vi "Simple Add.vi"(9 "Z":dbl, 10 "Y":dbl, 11 "X":dbl) -> (3 "Answer":dbl)   [LabVIEW 2016]
panel:
  # "Answer = 2x(X+Y+Z)"
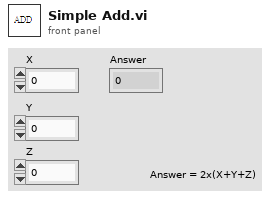
[diagram p1: front panel]
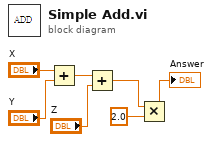
[diagram p0: block diagram]
diagram:
  n1 = Add(x="X", y="Y") -> (x+y=w5:dbl)
  n2 = Add(x=w5, y="Z") -> (x+y=w3:dbl)
  n3 = Multiply(x=w3, y=2.0) -> (x*y=→"Answer":dbl)
